vi "Slow_response_mean.vi"(4 "Index":i32, 5 "Block No":i32=1, 6 "Shift in":dbl[](array[numeric]) format="%.2f", 8 "U":dbl[](array[numeric]) format="%.2f") -> (0 "Shift out":dbl[](array[numeric]) format="%.2f", 3 "Results file string array":string[](array[string]))   [LabVIEW 2010]
uses:
  Globals/Meas_global.vi
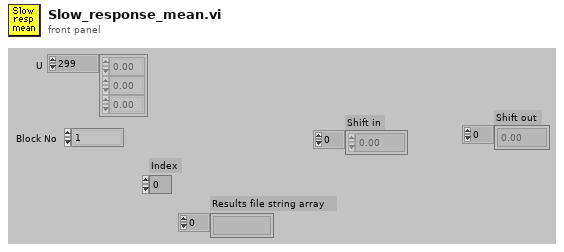
[diagram p1: front panel]
types:
  T1 = typedef "Velocity_cluster.ctl" = cluster{"Name":string, "U":dbl, "u^2":dbl, "u^3/(u^2)^(1.5)":dbl, "u^4/(u^2)^2 -3":dbl, "% u'/U":dbl, "Mean % Err":dbl, "u^4":dbl}
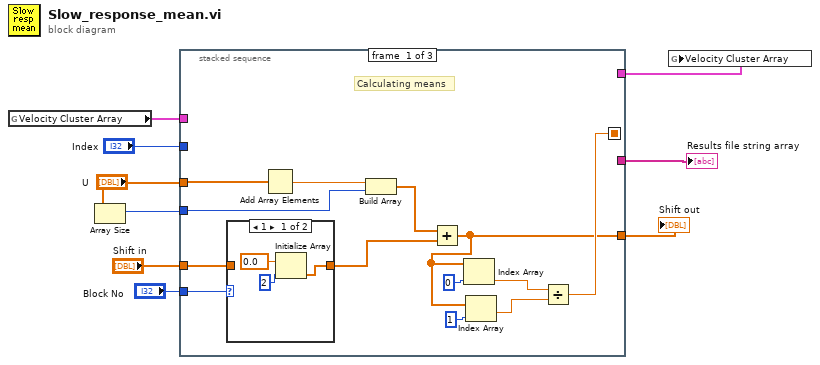
[diagram p0: block diagram]
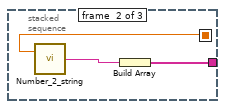
[diagram p3: hidden frame]
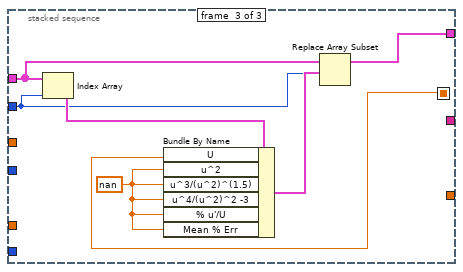
[diagram p4: hidden frame]
diagram:
  n1 = global read "Meas_global.vi" "Velocity Cluster Array"() -> (w7:T1[])
  n2 = Array Size(array="U") -> (size(s)=w4:i32)
  n3 = stacked-sequence {
    seq-local: [w22 _ _] -> [_ w28 w31]
    tunnel: "U" -> [w21 _ _]
    tunnel: [_ w29 _] -> w8
    tunnel: w7 -> [_ _ w34]
    tunnel: "Index" -> [_ _ w33]
    tunnel: [_ _ w32] -> w5
    tunnel: w4 -> [w19 _ _]
    tunnel: "Shift in" -> [w16 _ _]
    tunnel: "Block No" -> [w15 _ _]
    tunnel: [w10 _ _] -> w1
    frame #0 {
      # "Calculating means"
      n4 = case shown="1" w15 {
        tunnel: [w23 w26] -> w17
        tunnel: w16 -> [_ w26]
        frame 1 {
          n5 = Initialize Array(0.0 ("Element Data"), 2 ("Dimension Size")) -> (w23:dbl[])
        }
        frame 2, Default {
        }
      }
      n6 = Add Array Elements(numeric array=w21) -> (sum=w20:dbl)
      n7 = Build Array(w20, w19) -> (w18:dbl[])
      n8 = Add(x=w18, y=w17) -> (x+y=w10:dbl[])
      n9 = Index Array(array=w10, index=0 ("Index")) -> (element=w12:dbl)
      n10 = Index Array(array=w10, index=1 ("Index")) -> (element=w11:dbl)
      n11 = Divide(x=w12, y=w11) -> (x/y=w22:dbl)
    }
    frame #1 {
      n12 = call "Number_2_string.vi"("number"=w28) -> ("String"=w27:string)  [unwired: 1 in]
      n13 = Build Array(w27) -> (w29:string[])
    }
    frame #2 {
      w30 = nan ("u^3/(u^2)^(1.5)")
      n14 = Index Array(array=w34, index=w33) -> (element=w36:T1)
      n15 = Bundle By Name(cluster=w36, "U"=w31, "u^2"=w30, "u^3/(u^2)^(1.5)"=w30, "u^4/(u^2)^2 -3"=w30, "% u'/U"=w30, "Mean % Err"=w30) -> (w35:T1)
      n16 = Replace Array Subset(array=w34, new element=w35, index=w33) -> (w32:T1[])
    }
  }
  "Shift out" <- w1
  "Results file string array" <- w8
  n17 = global write "Meas_global.vi" "Velocity Cluster Array"(w5) -> ()
